vi "Read Config Binary.vi"(4 "Class Name is Included":bool, 6 "byte order (0:big-endian, network order)":T1(ring), 8 "error in (no error)":errorcluster, 10 "Binary":string, 11 "Abs_Type in":refnum<class "Abs_Type.lvclass">) -> (0 "error out":errorcluster, 2 "Remaining":string, 3 "Abs_Type out":refnum<class "Abs_Type.lvclass">)   [LabVIEW 2021, in "Abs_Type.lvclass"]
uses:
  Abs_Type.lvclass
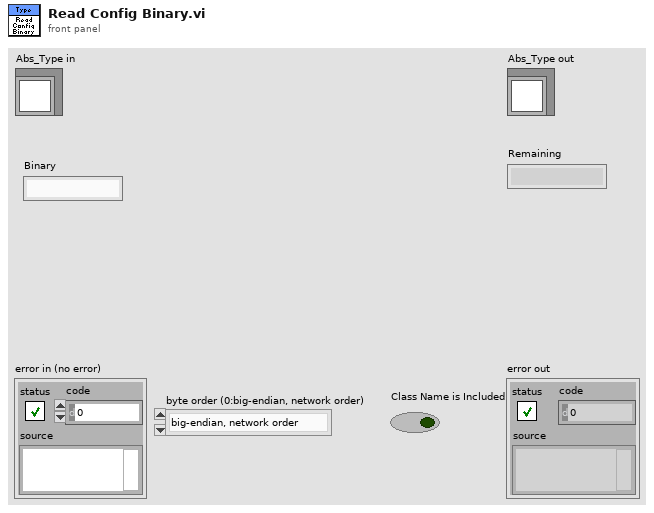
[diagram p1: front panel]
types:
  T1 = enum16{"big-endian, network order", "native, host order", "little-endian"}
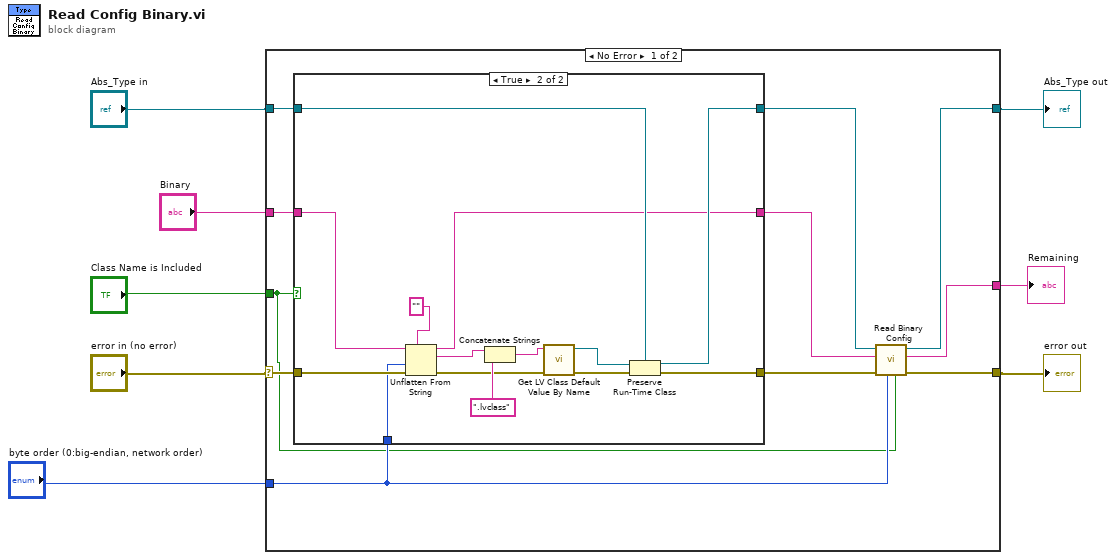
[diagram p0: block diagram]
diagram:
  n1 = case shown="No Error" "error in (no error)" {
    selector: "error in (no error)" -> [w19 w38]
    tunnel: [w15 w38] -> w6
    tunnel: [w12 w37] -> w5
    tunnel: "Abs_Type in" -> [w17 w37]
    tunnel: "Binary" -> [w18 _]
    tunnel: "byte order (0:big-endian, network order)" -> [w14 _]
    tunnel: "Class Name is Included" -> [w9 _]
    tunnel: [w10 _] -> w1
    frame No Error {
      n2 = case shown="True" w9 {
        tunnel: w19 -> [w22 w36]
        tunnel: w18 -> [w20 w35]
        tunnel: w14 -> [_ w34]
        tunnel: w17 -> [w21 w32]
        tunnel: [w21 w31] -> w13
        tunnel: [w22 w30] -> w16
        tunnel: [w20 w23] -> w11
        frame False {
        }
        frame True {
          n3 = Unflatten From String(type="", binary string=w35, byte order (0:big-endian, network order)=w34, error in (no error)=w36) -> (rest of the binary string=w23:string, value=w24:string, error out=w27:errorcluster)  [unwired: 1 in]
          n4 = Concatenate Strings(w24, ".lvclass" ("string")) -> (w29:string)
          n5 = call <vilib>:"Get LV Class Default Value By Name.vi"("error in (no error)"=w27, "class name"=w29) -> ("error out"=w26:errorcluster, "object"=w25:refnum<class>)  [unwired: 8 in]
          n6 = Preserve Run-Time Class(object in=w25, error in=w26, 2:w32) -> (object out=w31:refnum<class "Abs_Type.lvclass">, error out=w30:errorcluster)
        }
      }
      n7 = call-dynamic "Read Binary Config.vi"("Class Name is Included"=w9, "byte order (0:big-endian, network order)"=w14, "error in (no error)"=w16, "Binary"=w11, "Abs_Type in"=w13) -> ("error out"=w15:errorcluster, "Remaining"=w10:string, "Abs_Type out"=w12:refnum<class "Abs_Type.lvclass">)  [unwired: 4 in]
    }
    frame Error {
    }
  }
  "error out" <- w6
  "Abs_Type out" <- w5
  "Remaining" <- w1
